vi "Get Process VI.vi"(8 "error in (no error)":errorcluster, 11 "Plugin_UI in":refnum<class "Plugin_UI.lvclass">) -> (0 "error out":errorcluster, 2 "VI Refnum":refnum<vi>, 3 "Plugin_UI out":refnum<class "Plugin_UI.lvclass">)   [LabVIEW 2020, in "Plugin.lvlib" / "Plugin_UI.lvclass"]
doc: "Gets Plugin_UI Configuration VI reference."
uses:
  Plugin_UI.lvclass
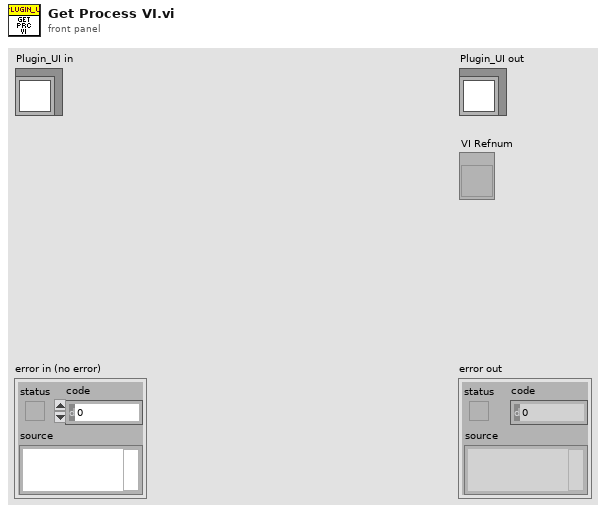
[diagram p1: front panel]
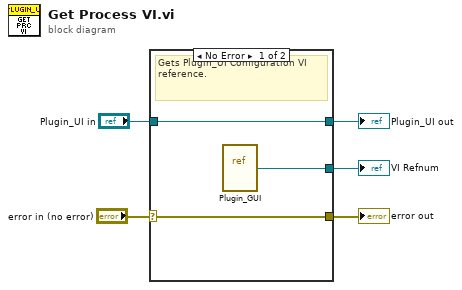
[diagram p0: block diagram]
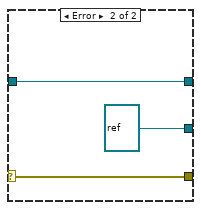
[diagram p2: hidden frame]
diagram:
  n1 = case shown="No Error" "error in (no error)" {
    selector: "error in (no error)" -> [w6 w9]
    tunnel: [w8 refnum<vi> refnum] -> w4
    tunnel: [w7 w10] -> w3
    tunnel: "Plugin_UI in" -> [w7 w10]
    tunnel: [w6 w9] -> w1
    frame No Error {
      # "Gets Plugin_UI Configuration VI reference."
      n2 = vi-ref "Plugin_GUI.vi"() -> (w8:refnum<vi>)
    }
    frame Error {
    }
  }
  "error out" <- w1
  "Plugin_UI out" <- w3
  "VI Refnum" <- w4
